vi "SelectRandomIndex.vi"(3 "Indices":i8[](array[numeric])) -> (1 "Selected Index":i8)   [LabVIEW 2020]
uses:
  <vilib>/numeric/Random Number (Range) I64.vi
  <vilib>/numeric/sub_Random U32.vi
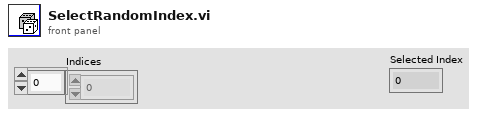
[diagram p1: front panel]
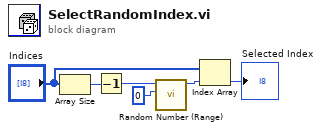
[diagram p0: block diagram]
diagram:
  n1 = Array Size(array="Indices") -> (size(s)=w6:i32)
  n2 = Decrement(x=w6) -> (x-1=w1:i32)
  n3 = call-poly <vilib>:"Random Number (Range).vi"("lower bound (-100)"=0, "upper bound (100)"=w1) -> ("number"=w4:i64)  [unwired: 9 in]
  n4 = Index Array(array="Indices", index=w4) -> (element=→"Selected Index":i8)
